vi "AcquisizioneDati.vi"(6 "error in":errorcluster, 7 "number of samples per channel":i32=100, 8 "task/channels in":refnum<k21>) -> (0 "Z-Signal Waveform":dynamicdata(graph), 1 "error out":errorcluster, 2 "Y-Signal Waveform":dynamicdata(graph), 3 "X-Signal Waveform":dynamicdata(graph), 4 "task out":refnum<k21>, 5 "3-Signal Waveform":waveform(dbl)[](graph))   [LabVIEW 2021]
uses:
  <vilib>/DAQmx/read.llb/DAQmx Read (Analog 1D Wfm NChan NSamp).vi
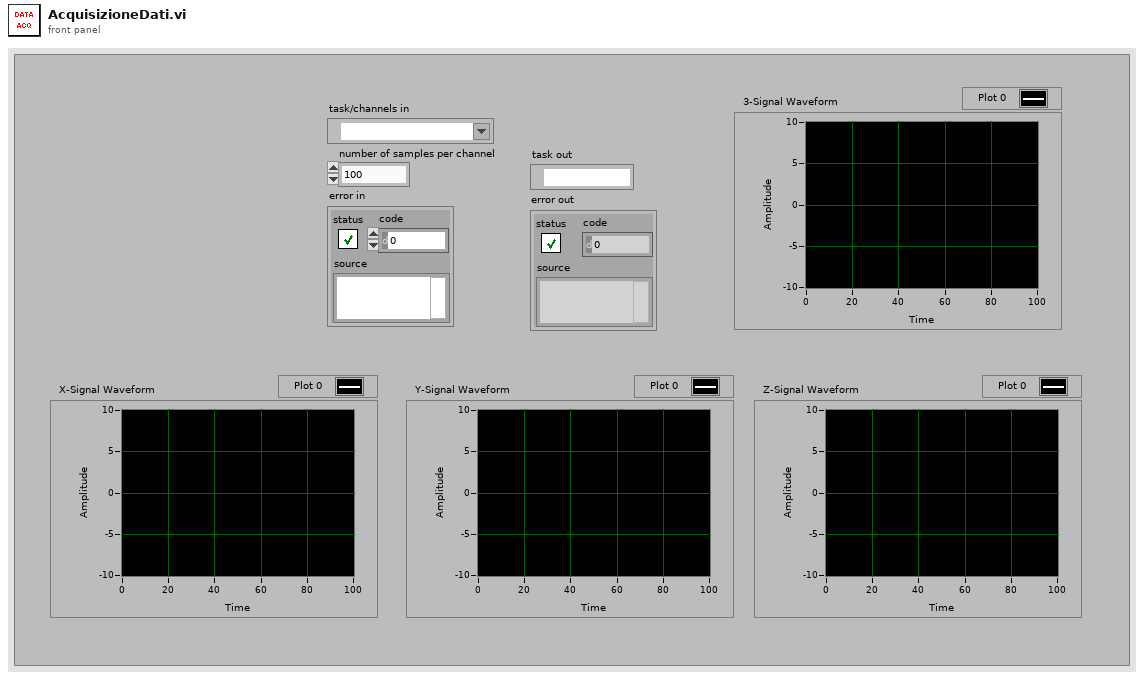
[diagram p1: front panel]
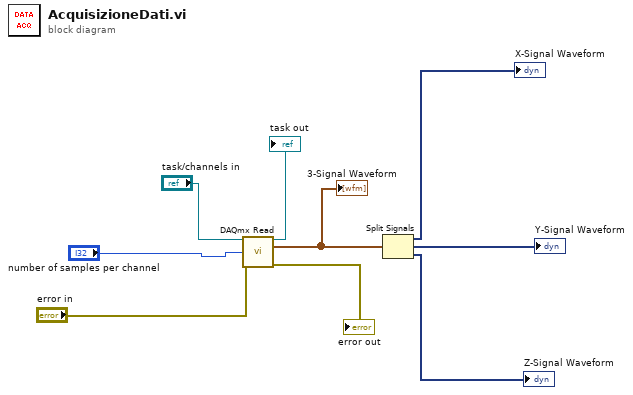
[diagram p0: block diagram]
diagram:
  n1 = call-poly <vilib>:"DAQmx Read.vi"("task/channels in"="task/channels in", "number of samples per channel"="number of samples per channel", "error in"="error in") -> ("task out"=→"task out":refnum<k21>, "data"=w6:waveform(dbl)[], "error out"=→"error out":errorcluster)  [unwired: 10 in]
  "3-Signal Waveform" <- w6
  n2 = Split Signals(w6) -> (→"X-Signal Waveform":dynamicdata, →"Y-Signal Waveform":dynamicdata, →"Z-Signal Waveform":dynamicdata)  [unwired: 3 in]
